vi "VISA_Write+Read.vi"(5 "NumRead":i32=1, 7 "Read? (T)":bool=TRUE, 8 "error in (no error)":errorcluster, 10 "Write Buffer":string, 11 "VISA resource name":refnum<visa-resource-name>) -> (0 "error out":errorcluster, 2 "readout":string, 3 "VISA resource name out":refnum<visa-resource-name>)   [LabVIEW 2014, in "GRBLMotionCore.lvlib"]
doc: "This Utility VI is a wrapper which writes to the instrument and reads the response. This VI is intended to be used as a private VI and altering it could cause several public VI's to operate incorrectly."
uses:
  <instrlib>/GRBL/GRBLMotionCore.lvlib
panel:
  out "appended array 2":string[](array[string])
  out "appended array":string[](array[string])
  out "s? t:f":string
  out "read buffer":string
  out "Com failure Cummulate":i32
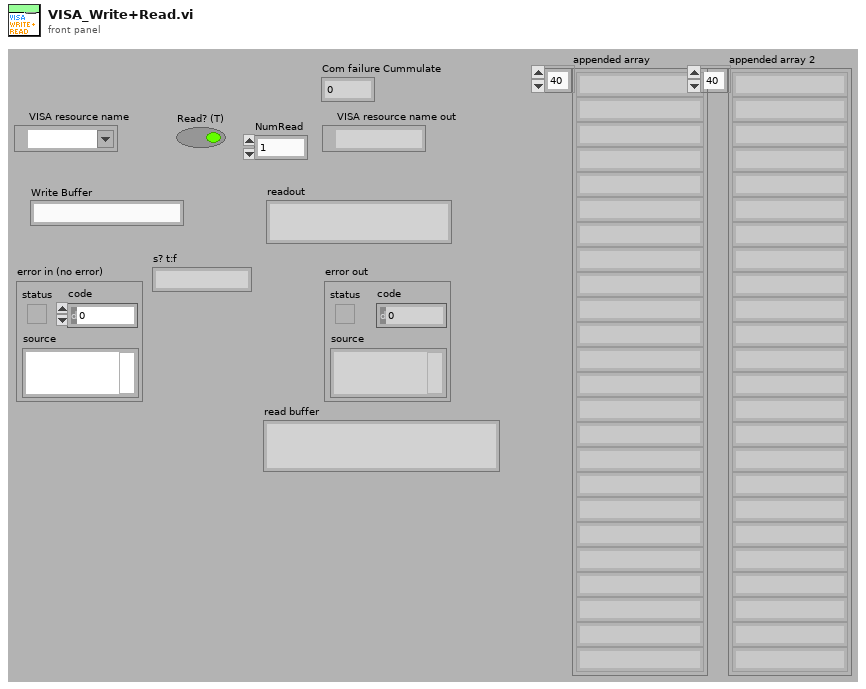
[diagram p1: front panel]
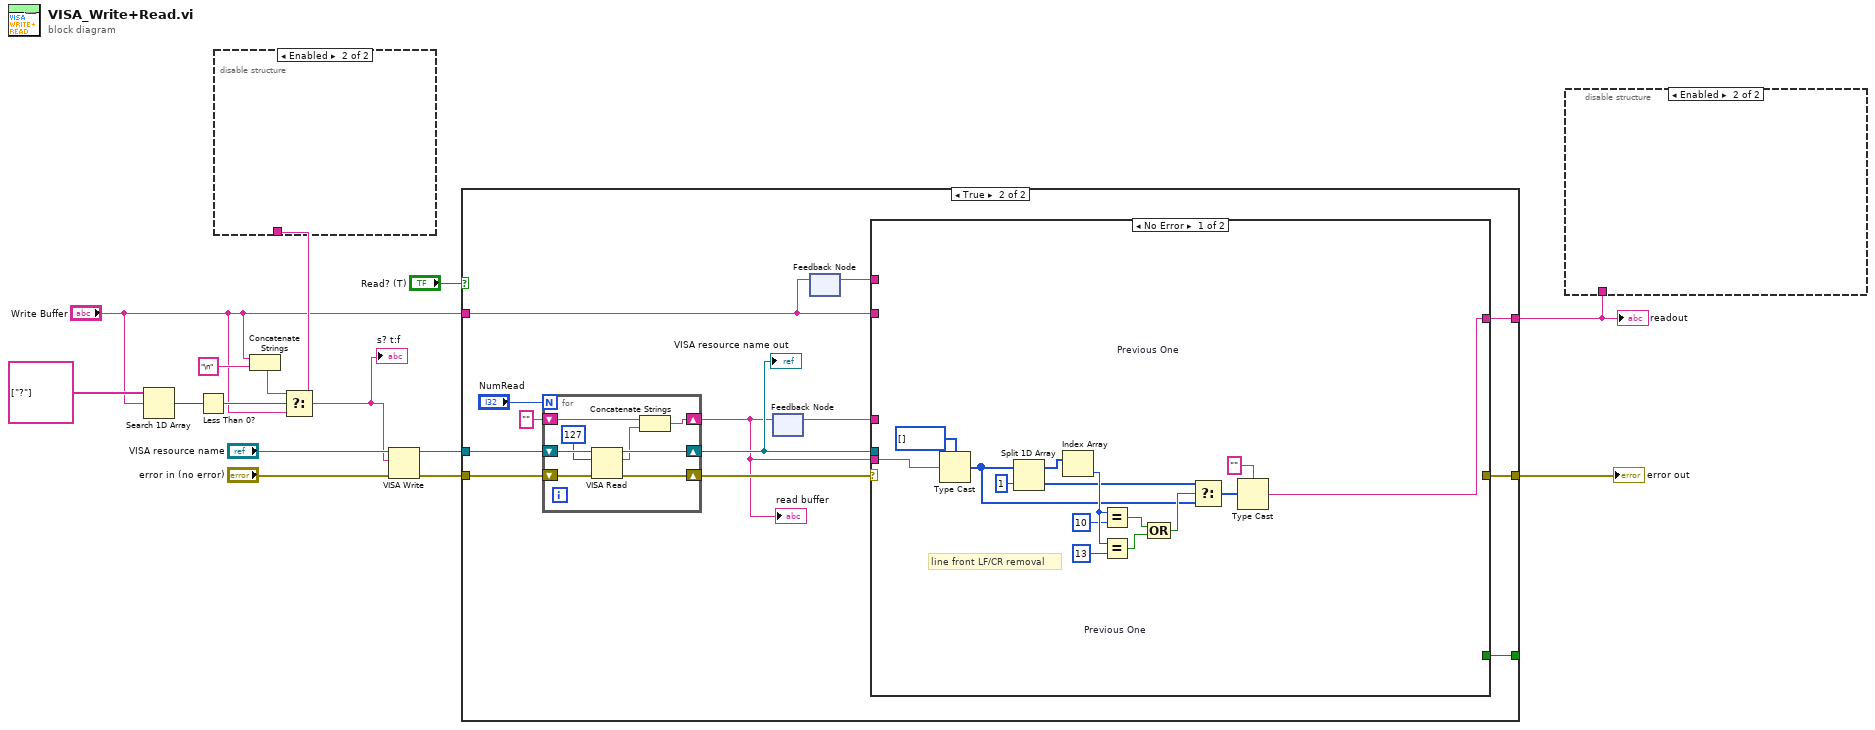
[diagram p0: block diagram]
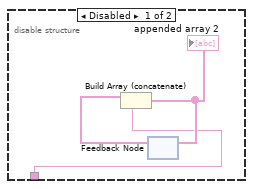
[diagram p2: hidden frame]
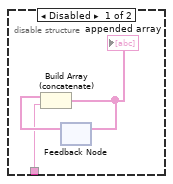
[diagram p3: hidden frame]
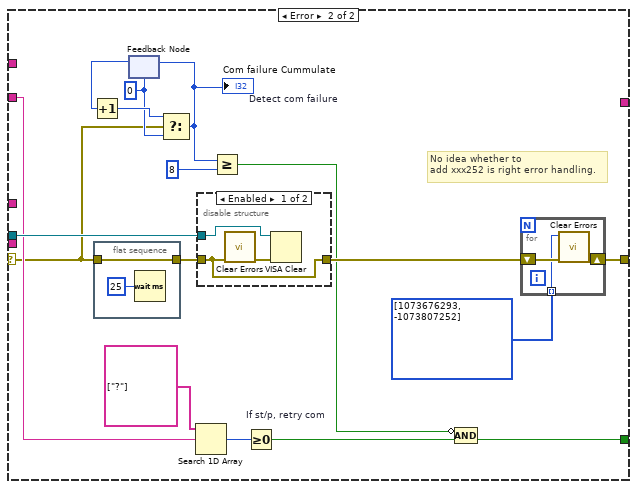
[diagram p5: hidden frame]
diagram:
  n1 = Search 1D Array(1D array=string[] ["?"], element="Write Buffer") -> (index of element=w1:i32)  [unwired: 1 in]
  n2 = Less Than 0?(x=w1) -> (x < 0?=w9:bool)
  n3 = Concatenate Strings("Write Buffer", "\n") -> (w11:string)
  n4 = Select(t=w11, s=w9, f="Write Buffer") -> (s? t:f=w7:string)
  "s? t:f" <- w7
  n5 = disable-structure shown="Enabled" {
    disable-tunnel: w7 -> [w15 _]
    frame Disabled {
      n6 = feedback #1() -> (w17:string[])  [unwired: 1 in]
      n7 = Build Array (concatenate)(w17, w15) -> (w16:string[])
      "appended array" <- w16
      n8 = feedback-in #1(w16) -> ()
    }
    frame Enabled {
    }
  }
  n9 = VISA Write(VISA resource name="VISA resource name", write buffer=w7, error in (no error)="error in (no error)") -> (VISA resource name out=w6:refnum<visa-resource-name>, error out=w5:errorcluster)  [unwired: 1 out]
  n10 = case shown="True" "Read? (T)" {
    tunnel: w6 -> [_ w24]
    tunnel: w5 -> [w18 w25]
    tunnel: "Write Buffer" -> [_ w30]
    tunnel: [w18 w28] -> w10
    tunnel: [_ w27] -> w8
    tunnel: [_ w26] -> _
    frame False {
    }
    frame True {
      n11 = for {
        N: "NumRead" -> [_]
        shift-right: [w37] -> w23
        shift-left: w24 -> [w38]
        shift-right: [w36] -> w22
        shift-left: w25 -> [w39]
        shift-right: [w33] -> w20
        shift-left: "" -> [w32]
        n12 = VISA Read(VISA resource name=w38, byte count=u32 127, error in (no error)=w39) -> (VISA resource name out=w37:refnum<visa-resource-name>, read buffer=w34:string, error out=w36:errorcluster)  [unwired: 1 out]
        n13 = Concatenate Strings(w32, w34) -> (w33:string)
      }
      "VISA resource name out" <- w23
      "read buffer" <- w20
      n14 = feedback #2 "Previous One"() -> (w29:string)  [unwired: 1 in]
      n15 = feedback-in #2(w20) -> ()
      n16 = feedback-in #3(w30) -> ()
      n17 = feedback #3 "Previous One"() -> (w31:string)  [unwired: 1 in]
      n18 = case shown="No Error" w22 {
        selector: w22 -> [_ w57]
        tunnel: w20 -> [w40 _]
        tunnel: w30 -> [_ w65]
        tunnel: w23 -> [_ w71]
        tunnel: w31 -> [_ _]
        tunnel: w29 -> [_ _]
        tunnel: [_ w68] -> w28
        tunnel: [w41 _] -> w27
        tunnel: [_ w56] -> w26
        frame No Error {
          # "line front LF/CR removal"
          n19 = Type Cast(type=u8[] [], x=w40) -> (*(type *) &x=w44:u8[])
          n20 = Split 1D Array(array=w44, index=1) -> (first subarray=w49:u8[], second subarray=w45:u8[])
          n21 = Index Array(array=w49) -> (element=w48:u8)  [unwired: 1 in]
          n22 = Equal?(x=w48, y=u8 10) -> (x = y?=w53:bool)
          n23 = Equal?(x=w48, y=u8 13) -> (x = y?=w54:bool)
          n24 = Compound Arithmetic op=OR(w53, w54) -> (w52:bool)
          n25 = Select(t=w45, s=w52, f=w44) -> (s? t:f=w43:u8[])
          n26 = Type Cast(type="" ("read buffer"), x=w43) -> (*(type *) &x=w41:string)
        }
        frame Error {
          w60 = 0
          # "No idea whether to \nadd xxx252 is right error handling."
          n27 = flat-sequence {
            tunnel: [w79] -> w70
            tunnel: w57 -> [w79]
            frame #0 {
              n28 = Wait (ms)(milliseconds to wait=u32 25) -> ()  [unwired: 1 out]
            }
          }
          n29 = feedback #4 "Detect com failure"(w60) -> (w61:i32)
          n30 = Increment(x=w61) -> (x+1=w62:i32)
          n31 = Select(t=w62, s=w57, f=w60) -> (s? t:f=w59:i32)
          "Com failure Cummulate" <- w59
          n32 = feedback-in #4(w59) -> ()
          n33 = Search 1D Array(1D array=string[] ["?"], element=w65) -> (index of element=w64:i32)  [unwired: 1 in]
          n34 = disable-structure shown="Enabled" {
            disable-tunnel: w71 -> [w77 _]
            disable-tunnel: w70 -> [w75 w78]
            disable-tunnel: [w75 w78] -> w67
            frame Enabled {
              n35 = call <vilib>:"Clear Errors.vi"("error in (no error)"=w75) -> ("error out"=w76:errorcluster)  [unwired: 5 in, 1 out]
              n36 = VISA Clear(VISA resource name=w77, error in (no error)=w76) -> ()  [unwired: 2 out]
            }
            frame Disabled {
            }
          }
          n37 = Greater Or Equal?(x=w59, y=8) -> (x >= y?=w55:bool)
          n38 = Greater Or Equal To 0? "If st/p, retry com"(x=w64) -> (x >= 0?=w63:bool)
          n39 = Compound Arithmetic op=AND(invert w55, w63) -> (w56:bool)
          n40 = for {
            shift-right: [w73] -> w68
            shift-left: w67 -> [w74]
            tunnel: i32[] [1073676293, -1073807252] -> [w72] mode=indexing
            n41 = call <vilib>:"Clear Errors.vi"("error in (no error)"=w74, "specific error code to clear (0: all)"=w72) -> ("error out"=w73:errorcluster)  [unwired: 4 in, 1 out]
          }
        }
      }
    }
  }
  "error out" <- w10
  "readout" <- w8
  n42 = disable-structure shown="Enabled" {
    disable-tunnel: w8 -> [w81 _]
    frame Disabled {
      n43 = feedback #5() -> (w82:string[])  [unwired: 1 in]
      n44 = Build Array (concatenate)(w82, w81) -> (w83:string[])
      "appended array 2" <- w83
      n45 = feedback-in #5(w83) -> ()
    }
    frame Enabled {
    }
  }
